vi "Check_Traverse_move_Low_PN.vi"(0 "Current position":sgl[](array[numeric])=[0.0, 200.0, 40.0] format="%.2f", 1 "New Position":sgl[](array[numeric])=[0.0, 100.0, 40.0] format="%.2f", 2 "Traverse Active Parts":cluster{"X":bool, "XY":bool, "XYZ":bool}, 3 "Model       Roll      Pitch       Yaw (deg)":sgl[](array[numeric]) format="%#.2f", 4 "Traverse Name":string) -> (5 "Error Comments":string, 6 "Traverse collision part":cluster{"X":bool, "XY":bool, "XYZ":bool}, 7 "Collision":bool)   [LabVIEW 2020]
uses:
  Collision_Detection/Triangles/EnFlo specific/Collision Mode.ctl
  Route_mapping_global.vi
  Globals/Trav_pos_global.vi
  Globals/Constants_global.vi
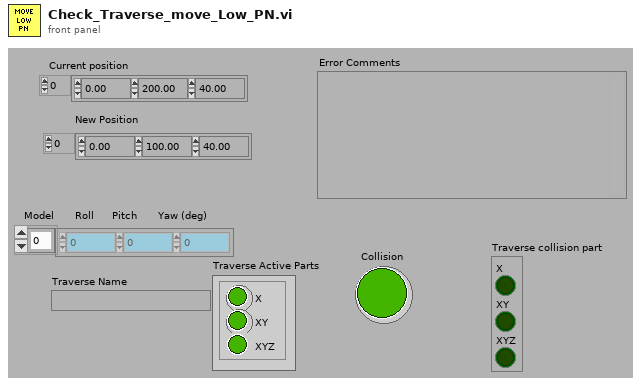
[diagram p1: front panel]
types:
  T1 = typedef "Box_size.ctl" = cluster{"Max":sgl, "Min":sgl}[]
  T2 = typedef "Collision Mode.ctl" = enum16{"Traverse - Tunnel", "Traverse - Model", "Traverse - Fixed objects", "Traverse - Traverse", "Traverse - All"}
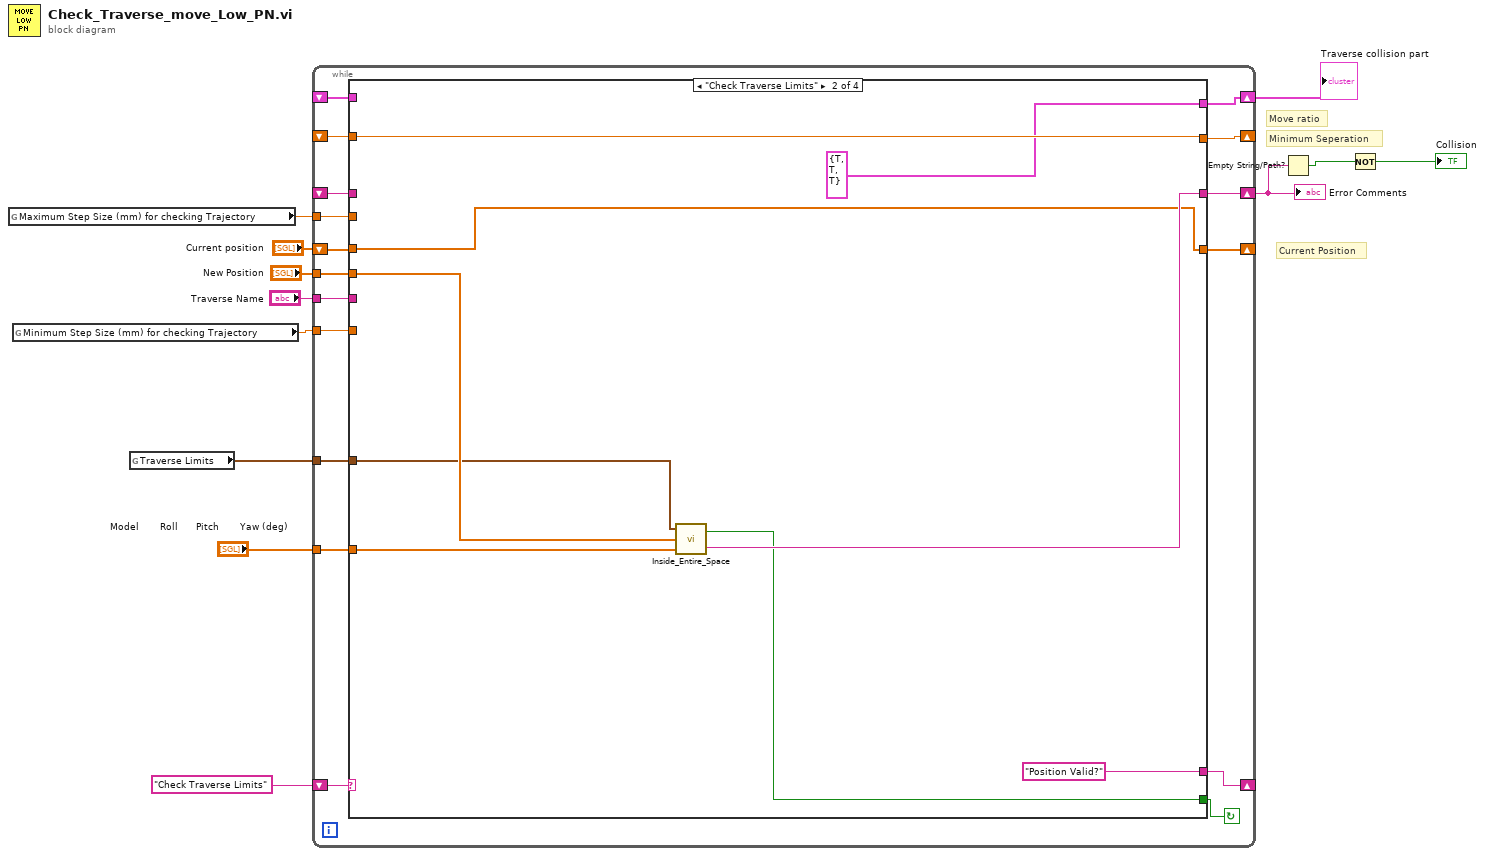
[diagram p0: block diagram]
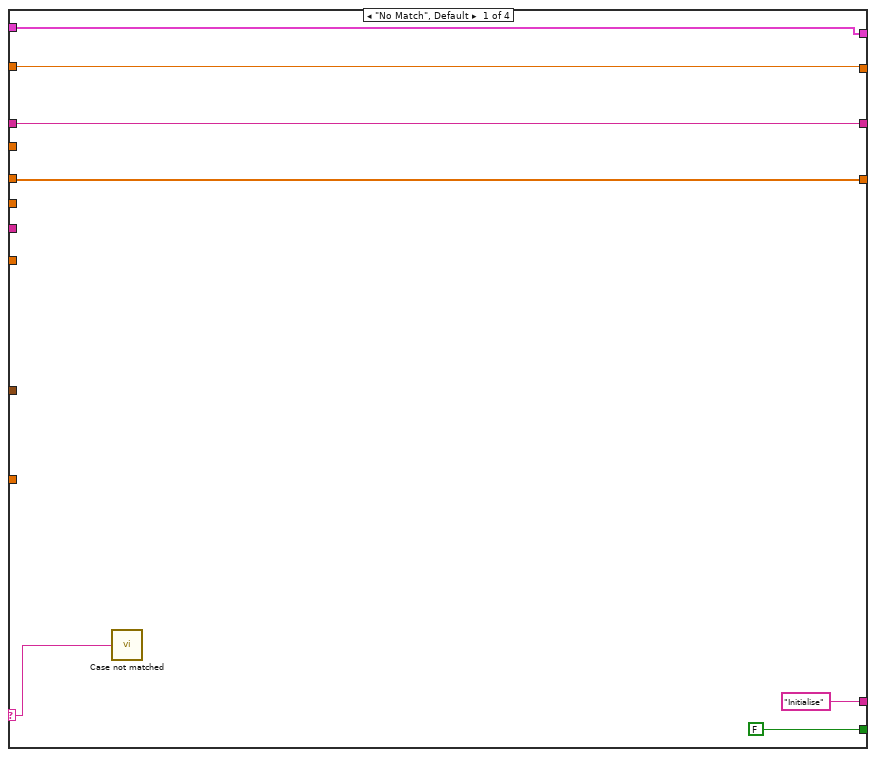
[diagram p2: hidden frame]
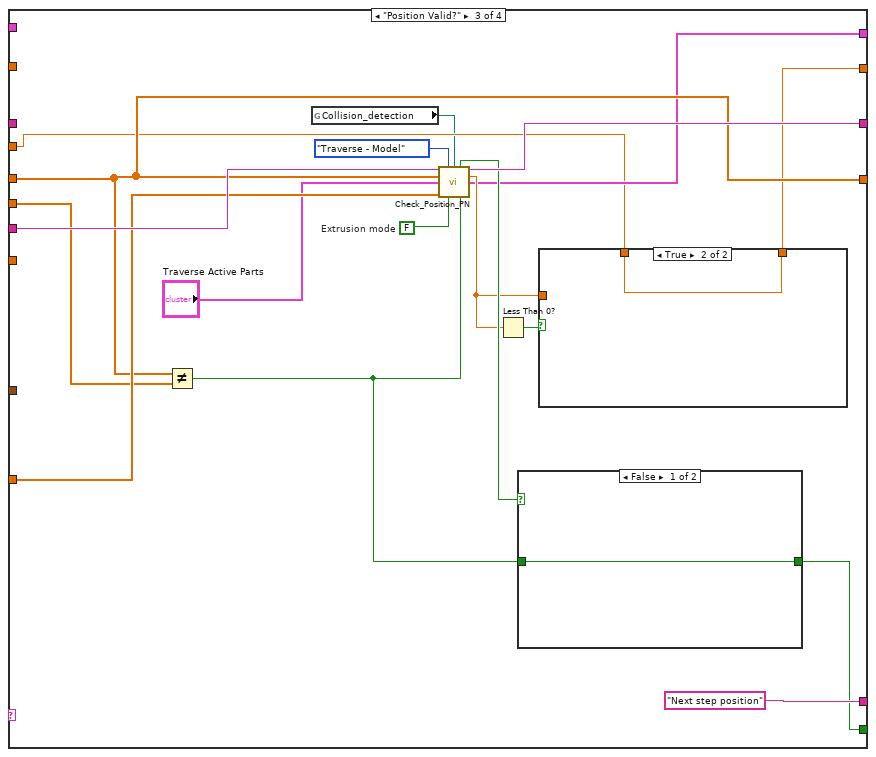
[diagram p3: hidden frame]
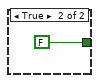
[diagram p5: hidden frame]
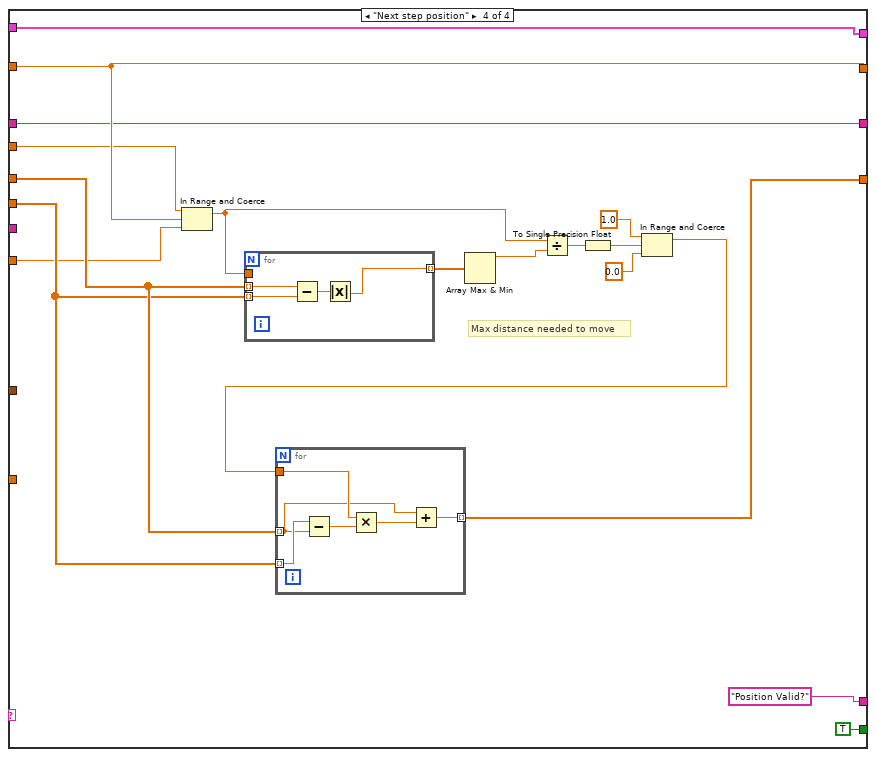
[diagram p6: hidden frame]
diagram:
  # "Current Position"
  # "Move ratio"
  # "Minimum Seperation"
  n1 = global read "Trav_pos_global.vi" "Maximum Step Size (mm) for checking Trajectory"() -> (w3:sgl)
  n2 = global read "Trav_pos_global.vi" "Minimum Step Size (mm) for checking Trajectory"() -> (w1:sgl)
  n3 = global read "Route_mapping_global.vi" "Traverse Limits"() -> (w9:T1)
  n4 = while {
    shift-left: "Check Traverse Limits" -> [w22]
    shift-right: [w29] -> _
    shift-right: [w26] -> w6
    shift-left: _ -> [w27]
    tunnel: "New Position" -> [w25]
    tunnel: "Traverse Name" -> [w24]
    tunnel: "Model       Roll      Pitch       Yaw (deg)" -> [w23]
    tunnel: w9 -> [w21]
    shift-right: [w20] -> _
    shift-left: _ -> [w19]
    shift-right: [w17] -> _
    shift-left: "Current position" -> [w18]
    tunnel: w3 -> [w16]
    shift-right: [w15] -> w2
    shift-left: _ -> [w14]
    tunnel: w1 -> [w13]
    stop <- w28 continue-if-true
    n5 = case shown="\"Check Traverse Limits\"" w22 {
      selector: w22 -> [w30 _ _ _]
      tunnel: [FALSE w42 w58 TRUE ("Box Inside")] -> w28
      tunnel: ["Initialise" "Position Valid?" "Next step position" "Position Valid?"] -> w29
      tunnel: w27 -> [w34 _ _ w77]
      tunnel: [w34 w44 w60 w77] -> w26
      tunnel: w18 -> [w32 w38 w57 w80]
      tunnel: w25 -> [_ w41 w56 w79]
      tunnel: w24 -> [_ _ w62 _]
      tunnel: w23 -> [_ w45 w61 _]
      tunnel: w21 -> [_ w40 _ _]
      tunnel: [w33 w39 w52 w82] -> w20
      tunnel: w19 -> [w33 w39 _ w82]
      tunnel: [w32 w38 w57 w78] -> w17
      tunnel: w16 -> [_ _ w48 w70]
      tunnel: [w31 cluster{"X":bool, "XY":bool, "XYZ":bool} {"X"=TRUE, "XY"=TRUE, "XYZ"=TRUE} ("Traverse collision part") w50 w69] -> w15
      tunnel: w14 -> [w31 _ _ w69]
      tunnel: w13 -> [_ _ _ w68]
      frame "No Match", Default {
        n6 = call "Case not matched.vi"("Case Name not Matched"=w30) -> ()
      }
      frame "Check Traverse Limits" {
        n7 = call "Inside_Entire_Space.vi"("Model       Roll      Pitch       Yaw (deg)"=w45, "Current Position"=w41, "Envelope"=w40) -> ("Error Comments"=w44:string, "Box Inside"=w42:bool)  [unwired: 1 in]
      }
      frame "Position Valid?" {
        w54 = FALSE  # Extrusion mode
        n8 = Not Equal?(x=w57, y=w56) -> (x != y?=w46:bool)
        n9 = global read "Constants_global.vi" "Collision_detection"() -> (w47:path)
        n10 = call "Check_Position_PN.vi"("Traverse Name"=w62, "Collision mode"=Collision_Mode."Traverse - Model", "Collision_detection"=w47, "Position to check"=w57, "Traverse Active Parts"="Traverse Active Parts", "Model Rotation (deg)"=w61, "Extrusion mode"=w54, "Get minimum separation within look-out sphere"=w46) -> ("Collision"=w59:bool, "Error Comments"=w60:string, "Minimum separation"=w51:sgl, "Traverse collision part"=w50:cluster{"X":bool, "XY":bool, "XYZ":bool})  [unwired: 3 in, 1 out]
        n11 = Less Than 0?(x=w51) -> (x < 0?=w53:bool)
        n12 = case shown="False" w59 {
          tunnel: [w66 FALSE] -> w58
          tunnel: w46 -> [w66 _]
          frame False {
          }
          frame True {
          }
        }
        n13 = case shown="True" w53 {
          tunnel: [w64 w65] -> w52
          tunnel: w51 -> [w64 _]
          tunnel: w48 -> [_ w65]
          frame False {
          }
          frame True {
          }
        }
      }
      frame "Next step position" {
        # "Max distance needed to move"
        n14 = In Range and Coerce(upper limit=w70, x=w82, lower limit=w68) -> (coerced(x)=w85:sgl)  [unwired: 1 out]
        n15 = for {
          tunnel: w80 -> [w95] mode=indexing
          tunnel: w79 -> [w94] mode=indexing
          tunnel: w85 -> [_]
          tunnel: [w92] -> w83 mode=indexing
          n16 = Subtract(x=w95, y=w94) -> (x-y=w93:sgl)
          n17 = Absolute Value(x=w93) -> (abs(x)=w92:sgl)
        }
        n18 = Array Max & Min(array=w83) -> (max value=w84:sgl)  [unwired: 3 out]
        n19 = Divide(x=w85, y=w84) -> (x/y=w81:sgl)
        n20 = To Single Precision Float(number=w81) -> (single precision float=w74:sgl)
        n21 = In Range and Coerce(upper limit=sgl 1.0, x=w74, lower limit=sgl 0.0) -> (coerced(x)=w71:sgl)  [unwired: 1 out]
        n22 = for {
          tunnel: w79 -> [w91] mode=indexing
          tunnel: w80 -> [w87] mode=indexing
          tunnel: w71 -> [w89]
          tunnel: [w86] -> w78 mode=indexing
          n23 = Subtract(x=w91, y=w87) -> (x-y=w90:sgl)
          n24 = Multiply(x=w89, y=w90) -> (x*y=w88:sgl)
          n25 = Add(x=w87, y=w88) -> (x+y=w86:sgl)
        }
      }
    }
  }
  "Error Comments" <- w6
  "Traverse collision part" <- w2
  n26 = Empty String/Path?(string/path=w6) -> (empty?=w5:bool)
  n27 = Not(x=w5) -> (.not. x?=→"Collision":bool)
